vi "FTW-TestStep-Base_TestExecInbox_Get.vi"(8 "error in (no error)":errorcluster, 11 "FTW-TestStep-Base In":refnum<class "FTW-TestStep-Base.lvclass">) -> (0 "error out":errorcluster, 2 "Test Exec Inbox":string, 3 "FTW-TestStep-Base Out":refnum<class "FTW-TestStep-Base.lvclass">)   [LabVIEW 2015, in "FTW-TestStep-Base.lvclass"]
uses:
  FTW-TestStep-Base.lvclass
  FTW-TestStep-Base.lvclass/FTW-TestStep-Base.ctl
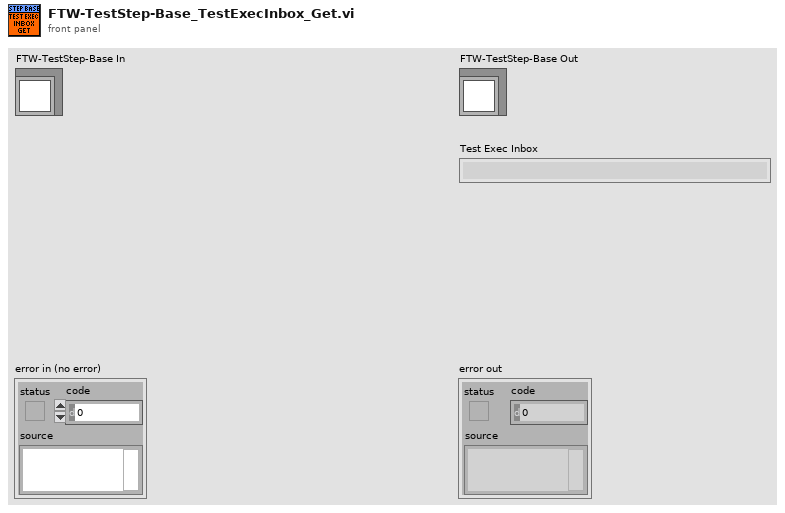
[diagram p1: front panel]
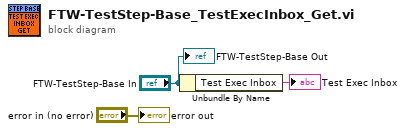
[diagram p0: block diagram]
diagram:
  n1 = Unbundle By Name("FTW-TestStep-Base In") -> ("Test Exec Inbox"=→"Test Exec Inbox":string)
  "error out" <- "error in (no error)"
  "FTW-TestStep-Base Out" <- "FTW-TestStep-Base In"
